vi "_TreeItem.Property.Get.Dictionary.Info.vi"(8 "error in (no error)":errorcluster, 11 "DictionaryProperty":refnum<k24>) -> (0 "error out":errorcluster, 1 "Keys":string[](array[string]), 2 "DictionaryType":string, 3 "DictionaryProperty out":refnum<k24>)   [LabVIEW 2016, in "Advanced System Definition.lvlib"]
uses:
  SysDef API/Advanced System Definition.lvlib
  NationalInstruments.VeriStand.SystemStorage
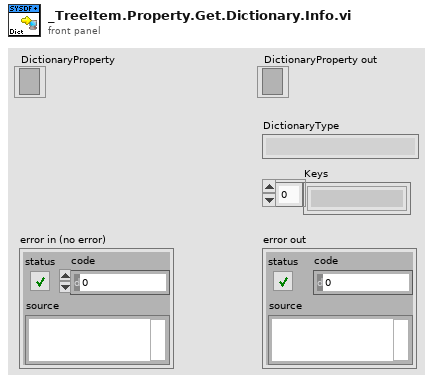
[diagram p1: front panel]
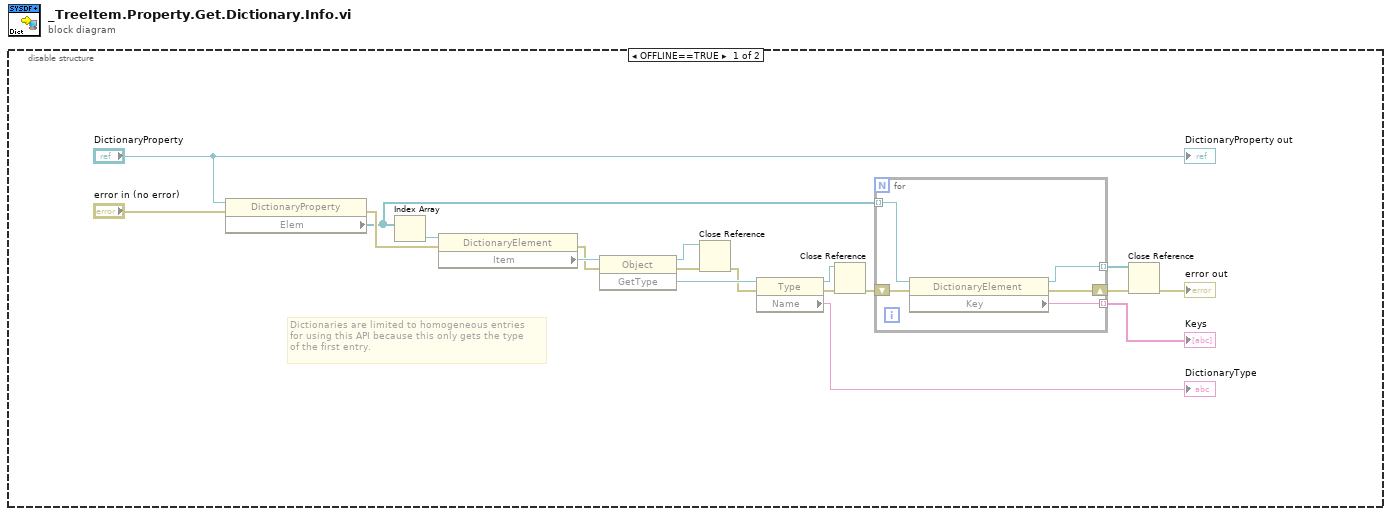
[diagram p0: block diagram]
diagram:
  n1 = disable-structure shown="OFFLINE==TRUE" {
    frame condition #0 {
      # "Dictionaries are limited to homogeneous entries\nfor using this API because this only gets the type\nof the first entry."
      n2 = property class="DictionaryProperty"(reference="DictionaryProperty", error in="error in (no error)") -> (error out=w15:errorcluster, "Elem"=w4:refnum<k24>[])  [unwired: 1 out]
      n3 = Index Array(array=w4) -> (element=w19:refnum<k24>)  [unwired: 1 in]
      n4 = property class="DictionaryElement"(reference=w19, error in=w15) -> (error out=w9:errorcluster, "Item"=w18:refnum<k24>)  [unwired: 1 out]
      n5 = invoke class="Object" method="GetType"(reference=w18, error in=w9) -> (reference out=w11:refnum<k24>, error out=w12:errorcluster, "GetType"=w17:refnum<k24>)  [unwired: 1 in]
      n6 = Close Reference(reference=w11, error in (no error)=w12) -> (error out=w10:errorcluster)
      n7 = property class="Type"(reference=w17, error in=w10) -> (reference out=w13:refnum<k24>, error out=w14:errorcluster, "Name"=→"DictionaryType":string)
      n8 = Close Reference(reference=w13, error in (no error)=w14) -> (error out=w3:errorcluster)
      n9 = for {
        tunnel: w4 -> [w24] mode=indexing
        tunnel: [w23] -> w5 mode=indexing
        shift-right: [w21] -> w2
        shift-left: w3 -> [w22]
        tunnel: [w20] -> w1 mode=indexing
        n10 = property class="DictionaryElement"(reference=w24, error in=w22) -> (reference out=w20:refnum<k24>, error out=w21:errorcluster, "Key"=w23:string)
      }
      "Keys" <- w5
      n11 = Close Reference(reference=w1, error in (no error)=w2) -> (error out=→"error out":errorcluster)
      "DictionaryProperty out" <- "DictionaryProperty"
    }
    frame condition #1 (active) {
    }
  }
